vi "Find Row Index from Property Name.vi"(8 "Error In":errorcluster, 10 "Property Name":string, 11 "Spreadsheet String Array":string[][](array[string])) -> (0 "Error Out":errorcluster, 2 "Row Index":i32, 3 "Spreadsheet String Array Out":string[][](array[string]))   [LabVIEW 2018]
doc: "Searches column 0 an array of strings (typically a text file the program has opened) for the search string specified and returns the row index."
uses:
  <vilib>/Utility/error.llb/Error Cluster From Error Code.vi
  <vilib>/ErrorRing/Error Ring.xnode
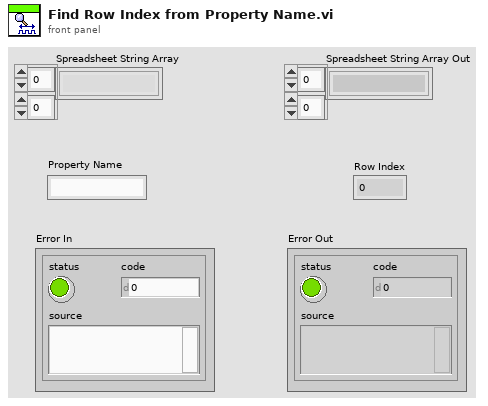
[diagram p1: front panel]
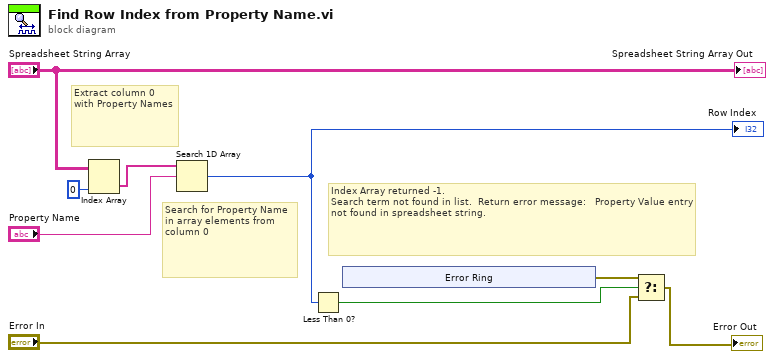
[diagram p0: block diagram]
diagram:
  # "Index Array returned -1.\nSearch term not found in list.  Return error message:   Property Value entry not found in spreadsheet string."
  # "Search for Property Name in array elements from column 0"
  # "Extract column 0 with Property Names"
  n1 = Index Array "Index Array"(array="Spreadsheet String Array", index (col)=0 ("disabled index (col)")) -> (element=w8:string[])  [unwired: 1 in]
  n2 = Search 1D Array(1D array=w8, element="Property Name") -> (index of element=w5:i32)  [unwired: 1 in]
  "Row Index" <- w5
  n3 = Less Than 0?(x=w5) -> (x < 0?=w4:bool)
  n4 = xnode "Error Ring"() -> ("error out"=w2:errorcluster)
  n5 = Select(t=w2, s=w4, f="Error In") -> (s? t:f=→"Error Out":errorcluster)
  "Spreadsheet String Array Out" <- "Spreadsheet String Array"
